vi "Simple Serial.vi"(7 "选项":enum16{"打开", "写入", "读取", "关闭"}(ring), 8 "error in":errorcluster, 9 "写入缓冲区":string, 10 "串口设置":T1={"波特率"=9600, "数据位"=8, "校验"=enum."None", "停止位"=10, "流控制"=0} {"流控制" items=["无"=0, "XON/XOFF"=1, "RTS/CTS"=2, "DTR/DSR"=4]; "停止位" items=["1.0"=10, "1.5"=15, "2.0"=20]; "数据位" min=5 max=8 step=1; "波特率" items=["75"=75, "110"=110, "134"=134, "150"=150, "300"=300, "600"=600, "1200"=1200, "1800"=1800, "2400"=2400, "4800"=4800, "7200"=7200, "9600"=9600, "14400"=14400, "19200"=19200, "28800"=28800, "38400"=38400, "56000"=56000, "57600"=57600, "115200"=115200, "128000"=128000, "230400"=230400]}, 11 "VISA资源名称":refnum<visa-resource-name>="COM1") -> (0 "error out":errorcluster, 2 "读取缓冲区":string, 3 "VISA resource name out":refnum<visa-resource-name>)   [LabVIEW 2017]
doc: "本范例执行串口读写操作。串口设置的参数必须匹配连接仪器或设备的参数。“VISA配置串口”VI可设置配置参数。前面板显示的控件可用于配置基本参数，如波特率、数据位和校验。VI会将VISA资源名称传递至其他VI以便执行相关操作。“VISA写入”函数将发送一个命令至串行设备，“VISA读取”函数将返回基于该命令的数据。“VISA关闭”函数可关闭该串行设备的引用。关闭引用十分重要，否则可能导致无法通过该端口进行进一步通信。"
uses:
  Serial - Settings.ctl
  <vilib>/Instr/_visa.llb/VISA Configure Serial Port (Instr).vi
panel:
  # "概述：演示使用VISA函数发送命令至串行仪器并读取响应。\n要求：NI-VISA驱动程序\n操作步骤：\n1.确保VISA资源名称为有效的串行设备。\n2.运行VI。\n3.如仪器识别了\"* IDN?\"命令，则应返回响应。"
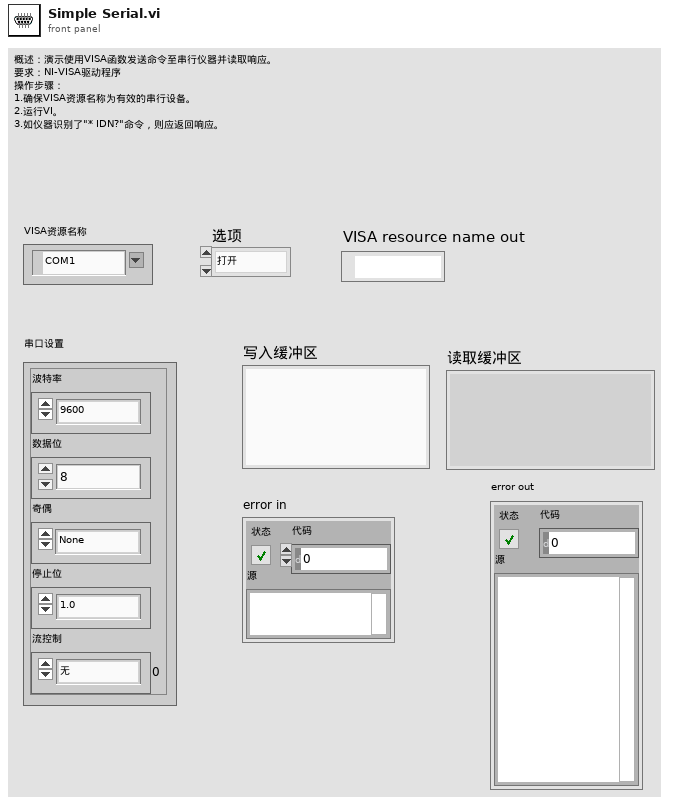
[diagram p1: front panel]
types:
  T1 = typedef "Serial - Settings.ctl" = cluster{"波特率":u32, "数据位":u16, "校验":enum16{"None", "Odd", "Even", "Mark", "Space"}, "停止位":u16, "流控制":u16}
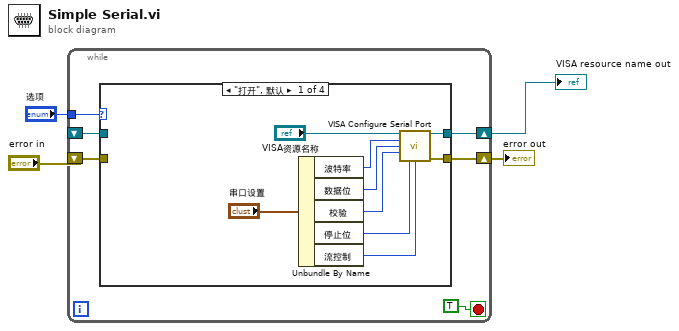
[diagram p0: block diagram]
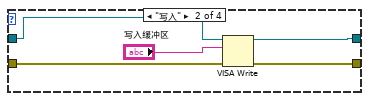
[diagram p2: hidden frame]
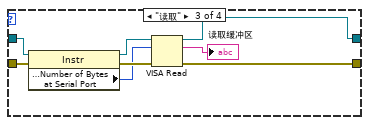
[diagram p3: hidden frame]
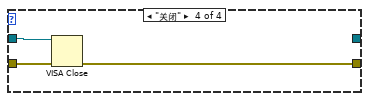
[diagram p4: hidden frame]
diagram:
  n1 = while {
    shift-right: [w9] -> w1
    shift-left: _ -> [w6]
    tunnel: "选项" -> [w7]
    shift-right: [w8] -> w2
    shift-left: "error in" -> [w5]
    stop <- TRUE stop-if-true
    n2 = case shown="\"打开\", 默认" w7 {
      tunnel: [w12 w23 w32 _] -> w9
      tunnel: [w11 w21 w31 w33] -> w8
      tunnel: w6 -> [_ w24 w29 w35]
      tunnel: w5 -> [_ w22 w27 w34]
      frame "打开", Default {
        n3 = Unbundle By Name("串口设置") -> ("波特率"=w15:u32, "数据位"=w16:u16, "校验"=w17:enum16{"None", "Odd", "Even", "Mark", "Space"}, "停止位"=w18:u16, "流控制"=w19:u16)
        n4 = call-poly "VISA Configure Serial Port"("VISA resource name"="VISA资源名称", "baud rate (9600)"=w15, "data bits (8)"=w16, "parity (0:none)"=w17, "stop bits (10: 1 bit)"=w18, "flow control (0:none)"=w19) -> ("VISA resource name out"=w12:refnum<visa-resource-name>, "error out"=w11:errorcluster)  [unwired: 3 in, 5 out]
      }
      frame "写入" {
        n5 = VISA Write(VISA resource name=w24, write buffer="写入缓冲区", error in (no error)=w22) -> (VISA resource name out=w23:refnum<visa-resource-name>, error out=w21:errorcluster)  [unwired: 1 out]
      }
      frame "读取" {
        n6 = property class="Instr"(reference=w29, error in=w27) -> (reference out=w28:refnum<visa-resource-name>, error out=w26:errorcluster, "Serial Settings:Number of Bytes at Serial Port"=w25:u32)
        n7 = VISA Read(VISA resource name=w28, byte count=w25, error in (no error)=w26) -> (VISA resource name out=w32:refnum<visa-resource-name>, read buffer=→"读取缓冲区":string, error out=w31:errorcluster)  [unwired: 1 out]
      }
      frame "关闭" {
        n8 = VISA Close(VISA resource name=w35, error in (no error)=w34) -> (error out=w33:errorcluster)
      }
    }
  }
  "error out" <- w2
  "VISA resource name out" <- w1
